vi "Create Disk Management Frames from Standard Out.vi"(11 "Standard Output":string) -> (2 "Writeable Drives Frame":variant, 3 "Disk Management Frame":variant)   [LabVIEW 2023]
uses:
  Type Definitions/Payload Class.ctl
  Type Definitions/Enum - System State.ctl
  Type Definitions/Disk State.ctl
  Type Definitions/Writeable Drives.ctl
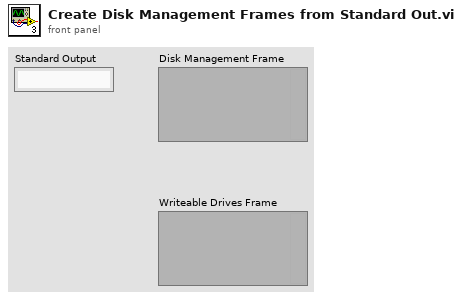
[diagram p1: front panel]
types:
  T1 = typedef "Enum - System State.ctl" = enum16{"System Time", "Telemetry TCP State", "Writeable Drive State", "Command TCP State", "Network Adapter State", "Discovery Engine State", "Disk State"}
  T2 = typedef "Writeable Drives.ctl" = cluster{"USB/SD Drives":path[], "Hard Drives":path[]}
  T3 = typedef "Payload Class.ctl" = enum16{"System State", "Parameters", "Metadata", "Software Monitor", "Data", "Commands"}
  T4 = typedef "Disk State.ctl" = cluster{"File System Name":string, "Total":sgl, "Available":sgl, "Used":sgl, "Path":string}
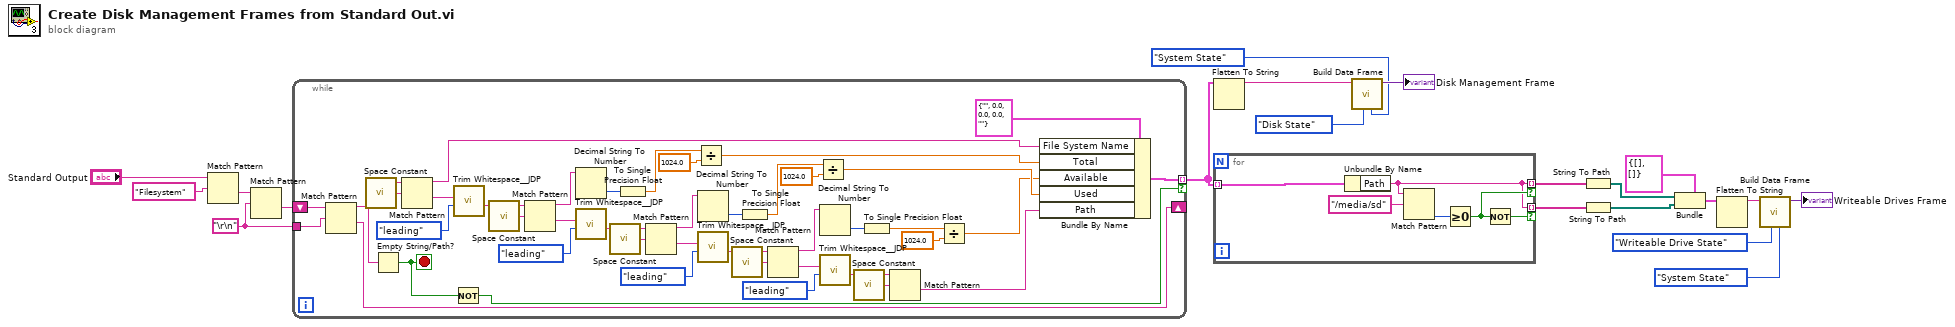
[diagram p0: block diagram]
diagram:
  w15 = "\r\n"
  n1 = Match Pattern(string="Standard Output", regular expression="Filesystem") -> (after substring=w14:string)  [unwired: 1 in, 3 out]
  n2 = Match Pattern(string=w14, regular expression=w15) -> (after substring=w16:string)  [unwired: 1 in, 3 out]
  n3 = while {
    tunnel: w15 -> [w62]
    tunnel: [w33] -> w2 mode=indexing if=w58
    shift-right: [w60] -> _
    shift-left: w16 -> [w61]
    stop <- w59 stop-if-true
    n4 = Match Pattern(string=w61, regular expression=w62) -> (before substring=w34:string, after substring=w60:string)  [unwired: 1 in, 2 out]
    n5 = call <vilib>:"Space Constant.vi"() -> ("String"=w39:string)
    n6 = Empty String/Path?(string/path=w34) -> (empty?=w59:bool)
    n7 = Match Pattern(string=w34, regular expression=w39) -> (before substring=w53:string, after substring=w31:string)  [unwired: 1 in, 2 out]
    n8 = Not(x=w59) -> (.not. x?=w58:bool)
    n9 = call <vilib>:"Trim Whitespace__JDP.vi"("Remove (leading and trailing)"=enum16{"leading", "trailing", "both"}."leading", "String in"=w31) -> ("String out"=w30:string)  [unwired: 5 in]
    n10 = call <vilib>:"Space Constant.vi"() -> ("String"=w40:string)
    n11 = Match Pattern(string=w30, regular expression=w40) -> (before substring=w44:string, after substring=w28:string)  [unwired: 1 in, 2 out]
    n12 = Decimal String To Number(string=w44) -> (number=w45:i32)  [unwired: 2 in, 1 out]
    n13 = call <vilib>:"Trim Whitespace__JDP.vi"("Remove (leading and trailing)"=enum16{"leading", "trailing", "both"}."leading", "String in"=w28) -> ("String out"=w27:string)  [unwired: 5 in]
    n14 = call <vilib>:"Space Constant.vi"() -> ("String"=w41:string)
    n15 = To Single Precision Float(number=w45) -> (single precision float=w46:sgl)
    n16 = Match Pattern(string=w27, regular expression=w41) -> (before substring=w49:string, after substring=w25:string)  [unwired: 1 in, 2 out]
    n17 = Divide(x=w46, y=sgl 1024.0) -> (x/y=w54:sgl)
    n18 = Decimal String To Number(string=w49) -> (number=w48:i32)  [unwired: 2 in, 1 out]
    n19 = call <vilib>:"Trim Whitespace__JDP.vi"("Remove (leading and trailing)"=enum16{"leading", "trailing", "both"}."leading", "String in"=w25) -> ("String out"=w24:string)  [unwired: 5 in]
    n20 = call <vilib>:"Space Constant.vi"() -> ("String"=w42:string)
    n21 = To Single Precision Float(number=w48) -> (single precision float=w47:sgl)
    n22 = Match Pattern(string=w24, regular expression=w42) -> (before substring=w52:string, after substring=w22:string)  [unwired: 1 in, 2 out]
    n23 = Divide(x=w47, y=sgl 1024.0) -> (x/y=w56:sgl)
    n24 = Decimal String To Number(string=w52) -> (number=w50:i32)  [unwired: 2 in, 1 out]
    n25 = call <vilib>:"Trim Whitespace__JDP.vi"("Remove (leading and trailing)"=enum16{"leading", "trailing", "both"}."leading", "String in"=w22) -> ("String out"=w21:string)  [unwired: 5 in]
    n26 = call <vilib>:"Space Constant.vi"() -> ("String"=w43:string)
    n27 = To Single Precision Float(number=w50) -> (single precision float=w51:sgl)
    n28 = Match Pattern(string=w21, regular expression=w43) -> (after substring=w57:string)  [unwired: 1 in, 3 out]
    n29 = Divide(x=w51, y=sgl 1024.0) -> (x/y=w55:sgl)
    n30 = Bundle By Name(cluster=T4 {"File System Name"="", "Total"=0.0, "Available"=0.0, "Used"=0.0, "Path"=""}, "File System Name"=w53, "Total"=w54, "Available"=w55, "Used"=w56, "Path"=w57) -> (w33:T4)
  }
  n31 = Flatten To String(anything=w2) -> (data string=w4:string)  [unwired: 3 in, 2 out]
  n32 = for {
    tunnel: w2 -> [w68] mode=indexing
    tunnel: [w64] -> w17 mode=indexing if=w65
    tunnel: [w64] -> w1 mode=indexing if=w63
    n33 = Unbundle By Name(w68) -> ("Path"=w64:string)
    n34 = Match Pattern(string=w64, regular expression="/media/sd") -> (offset past match=w66:i32)  [unwired: 1 in, 3 out]
    n35 = Greater Or Equal To 0?(x=w66) -> (x >= 0?=w65:bool)
    n36 = Not(x=w65) -> (.not. x?=w63:bool)
  }
  n37 = call "Build Data Frame.vi"("Payload Class (Data)"=Payload_Class."System State", "Payload ID (0)"=Enum_-_System_State."Disk State" ("System State"), "Payload (Empty String)"=w4) -> ("Frame"=→"Disk Management Frame":variant)  [unwired: 7 in, 1 out]
  n38 = String To Path(string=w17) -> (path=w18:path[])
  n39 = String To Path(string=w1) -> (path=w19:path[])
  n40 = Bundle(cluster=T2 {"USB/SD Drives"=[], "Hard Drives"=[]}, "USB/SD Drives"=w18, "Hard Drives"=w19) -> (w11:T2)
  n41 = Flatten To String(anything=w11) -> (data string=w8:string)  [unwired: 3 in, 2 out]
  n42 = call "Build Data Frame.vi"("Payload Class (Data)"=Payload_Class."System State", "Payload ID (0)"=Enum_-_System_State."Writeable Drive State" ("System State"), "Payload (Empty String)"=w8) -> ("Frame"=→"Writeable Drives Frame":variant)  [unwired: 7 in, 1 out]
